vi "Test Harness.vi"() -> ()   [LabVIEW 2017, in "Command Handler.lvlib"]
uses:
  Command Handler.lvlib
  Command Handler/Command Handler.lvclass
  C:/Program Files (x86)/National Instruments/LabVIEW 2017/vi.lib/ActorFramework/Actor/Actor.lvclass
  <vilib>/ActorFramework/Message Enqueuer/Message Enqueuer.lvclass/Message Enqueuer.ctl
  Command Parents/Command.lvclass
  Command Handler Messages/Load Command Msg/Load Command Msg.lvclass/Load Command Msg.ctl
  Command Handler Messages/Execute Command Msg/Execute Command Msg.lvclass/Execute Command Msg.ctl
  Command Handler Messages/Execute Loaded Commands Msg/Execute Loaded Commands Msg.lvclass/Execute Loaded Commands Msg.ctl
  <vilib>/ActorFramework/Message Enqueuer/Enqueue.vi
  <vilib>/ActorFramework/Stop Msg/Stop Msg.lvclass
  C:/Program Files (x86)/National Instruments/LabVIEW 2017/vi.lib/ActorFramework/Message/Message.lvclass
  Command Handler Messages/Load Command Msg/Load Command Msg.lvclass
  Command Handler Messages/Execute Command Msg/Execute Command Msg.lvclass
  Command Handler Messages/Execute Loaded Command Msg/Execute Loaded Command Msg.lvclass
  Command Handler Messages/Execute Loaded Commands Msg/Execute Loaded Commands Msg.lvclass
  <vilib>/ActorFramework/Message Priority Queue/Priority Enqueue.vi
  <vilib>/ActorFramework/Actor/Actor.lvclass
  Command Handler Messages/Return Events Msg/Return Events Msg.lvclass
panel:
  in  "Commands Folder":path
  out "Last Error Time":timestamp
  in  "Enable Command Handling":bool
  in  "Disable Command Handling":bool
  in  "Reload":bool
  out "Last Handler Error":errorcluster
  in  "Commands":string(combo)
  in  "Run Loaded Commands":bool
  in  "Front (T) Back (F)":bool
  in  "Run Next Loaded Command":bool
  in  "Execute Command":bool
  in  "Add Command":bool
  out "Completed Commands":string[](array[string])
  out "Commands Completed":i32
  out "Loaded Commands":string[](array[string])
  out "Commands Loaded":i32
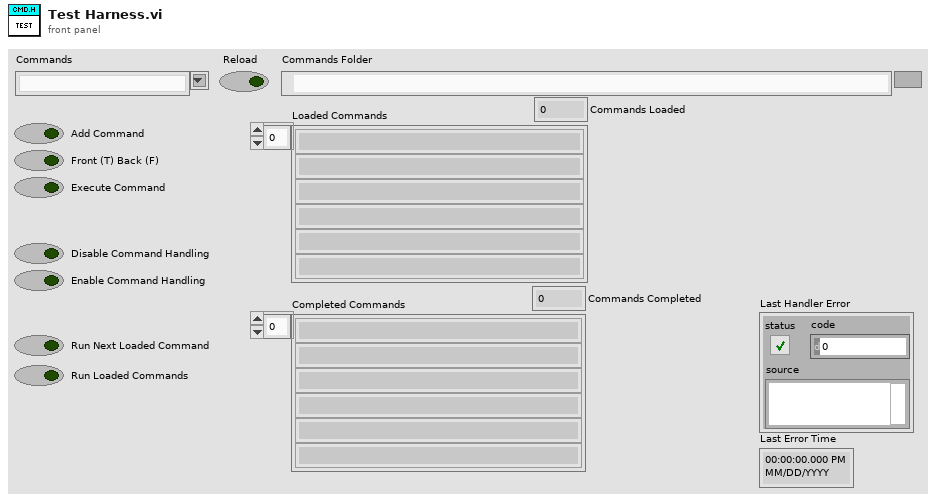
[diagram p1: front panel]
types:
  T1 = typedef "Command Handler.lvlib/Command Handler.lvclass/Event Cluster.ctl" = cluster{"Error Event":refnum<user-event>, "Command Done Event":refnum<user-event>, "Stopping Event":refnum<user-event>, "Data Update Event":refnum<user-event>}
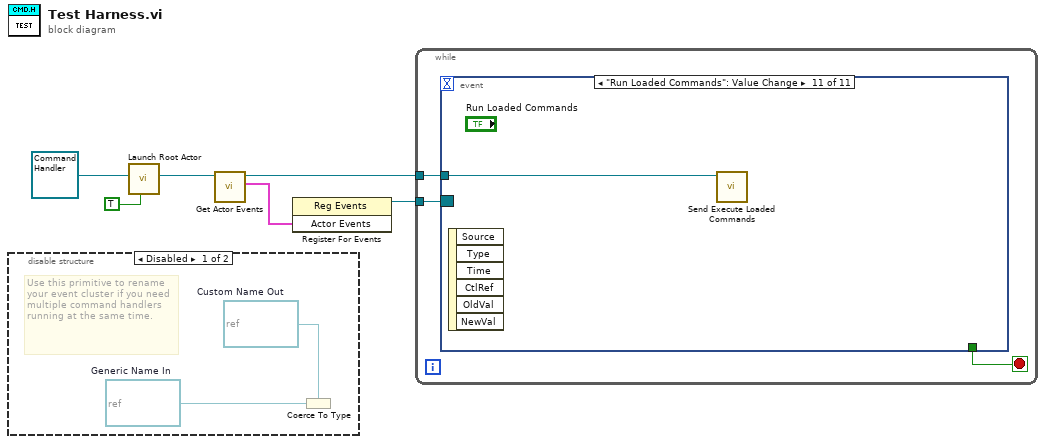
[diagram p0: block diagram]
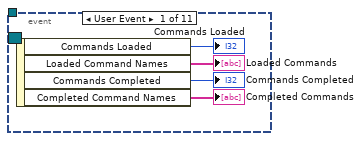
[diagram p3: hidden frame]
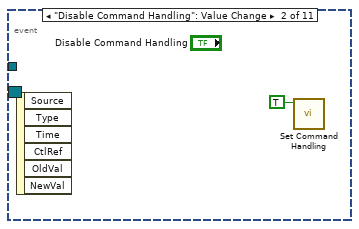
[diagram p4: hidden frame]
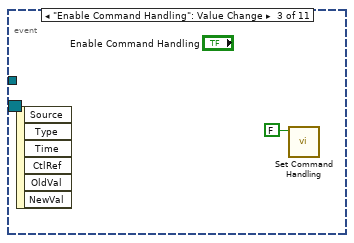
[diagram p5: hidden frame]
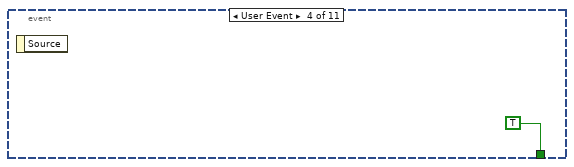
[diagram p6: hidden frame]
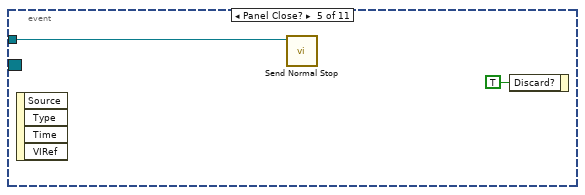
[diagram p7: hidden frame]
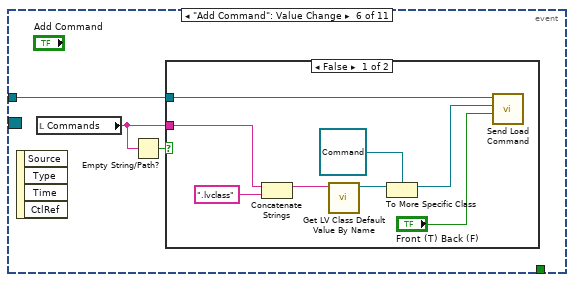
[diagram p8: hidden frame]
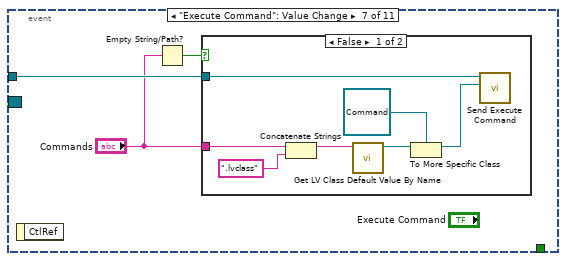
[diagram p10: hidden frame]
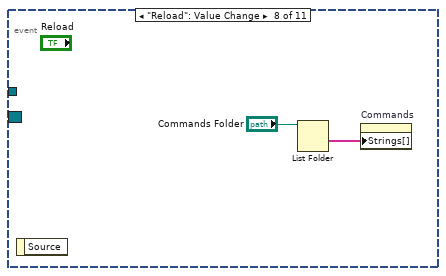
[diagram p12: hidden frame]
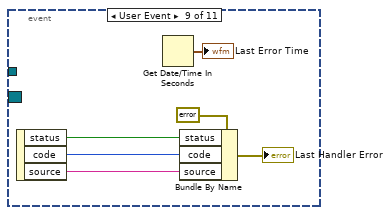
[diagram p13: hidden frame]
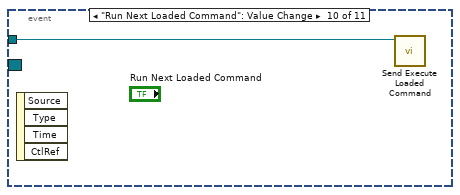
[diagram p14: hidden frame]
diagram:
  n1 = disable-structure shown="Disabled" {
    frame Disabled {
      w7 = refnum<user-event> refnum  # Custom Name Out
      w8 = refnum<user-event> refnum  # Generic Name In
      # "Use this primitive to rename your event cluster if you need multiple command handlers running at the same time."
      n2 = Coerce To Type(0:w8, 1:w7) -> ()  [unwired: 1 out]
    }
    frame Enabled {
    }
  }
  n3 = call <vilib>:"Launch Root Actor.vi"("Open Actor Core front panel? (F)"=TRUE, "Actor"=refnum<class "Command Handler.lvclass"> refnum ("Command Handler.lvlib:Command Handler.lvclass")) -> ("Actor's Enqueuer"=w1:refnum<class "Message Enqueuer.lvclass">)  [unwired: 8 in, 1 out]
  n4 = call "Get Actor Events.vi"("Message Enqueuer in"=w1) -> ("Actor Events"=w2:T1, "Message Enqueuer out"=w5:refnum<class "Message Enqueuer.lvclass">)  [unwired: 7 in, 2 out]
  n5 = register-events(w2) -> (reference out=w6:refnum<event-registration>)  [unwired: 2 in, 1 out]
  n6 = while {
    tunnel: w6 -> [w11]
    tunnel: w5 -> [w9]
    stop <- w10 stop-if-true
    n7 = event shown="[10] \"Run Loaded Commands\": Value Change" {
      selector: w11 -> [_ _ _ _ _ _ _ _ _ _ _]
      dyn-events: _ -> [_ _ _ _ _ _ _ _ _ _ _]
      timeout: _ -> [_ _ _ _ _ _ _ _ _ _ _]
      tunnel: [_ _ _ TRUE _ _ _ _ _ _ _] -> w10
      tunnel: w9 -> [_ _ _ _ w20 w23 w34 _ _ w50 w51]
      event User Event {
        n8 = event-data() -> ("Commands Loaded"=→"Commands Loaded":i32, "Loaded Command Names"=→"Loaded Commands":string[], "Commands Completed"=→"Commands Completed":i32, "Completed Command Names"=→"Completed Commands":string[])  [unwired: 1 in]
      }
      event "Disable Command Handling": Value Change {
        n9 = event-data() -> ()  [unwired: 1 in, 6 out]
        n10 = call "Set Command Handling.vi"("Disable Command Handling"=TRUE ("Command Handling Stopped")) -> ()  [unwired: 10 in, 1 out]
      }
      event "Enable Command Handling": Value Change {
        n11 = event-data() -> ()  [unwired: 1 in, 6 out]
        n12 = call "Set Command Handling.vi"("Disable Command Handling"=FALSE ("Command Handling Stopped")) -> ()  [unwired: 10 in, 1 out]
      }
      event User Event {
        n13 = event-data() -> ()  [unwired: 1 in, 1 out]
      }
      event Panel Close? {
        n14 = event-data() -> ()  [unwired: 1 in, 4 out]
        n15 = call <vilib>:"Send Normal Stop.vi"("Message Enqueuer"=w20) -> ()  [unwired: 10 in, 1 out]
        n16 = event-data("Discard?"=TRUE) -> ()  [unwired: 1 in, 1 out]
      }
      event "Add Command": Value Change {
        n17 = event-data() -> ()  [unwired: 1 in, 4 out]
        n18 = local read "Commands"() -> (w22:string)
        n19 = Empty String/Path?(string/path=w22) -> (empty?=w21:bool)
        n20 = case shown="False" w21 {
          tunnel: w23 -> [w31 _]
          tunnel: w22 -> [w24 _]
          frame False {
            n21 = Concatenate Strings(w24, ".lvclass" ("string")) -> (w26:string)
            n22 = call <vilib>:"Get LV Class Default Value By Name.vi"("class name"=w26) -> ("object"=w29:refnum<class>)  [unwired: 9 in, 1 out]
            n23 = To More Specific Class(target class=refnum<class "Command.lvclass"> refnum ("Command.lvclass"), reference=w29) -> (specific class reference=w28:refnum<class "Command.lvclass">)  [unwired: 1 in, 1 out]
            n24 = call "Send Load Command.vi"("Front (T) Back (F)"="Front (T) Back (F)", "Command In"=w28, "Message Enqueuer"=w31) -> ()  [unwired: 7 in, 2 out]
          }
          frame True {
          }
        }
      }
      event "Execute Command": Value Change {
        n25 = event-data() -> ()  [unwired: 1 in, 1 out]
        n26 = Empty String/Path?(string/path="Commands") -> (empty?=w33:bool)
        n27 = case shown="False" w33 {
          tunnel: w34 -> [w41 _]
          tunnel: "Commands" -> [w35 _]
          frame False {
            n28 = Concatenate Strings(w35, ".lvclass" ("string")) -> (w38:string)
            n29 = call <vilib>:"Get LV Class Default Value By Name.vi"("class name"=w38) -> ("object"=w40:refnum<class>)  [unwired: 9 in, 1 out]
            n30 = To More Specific Class(target class=refnum<class "Command.lvclass"> refnum ("Command.lvclass"), reference=w40) -> (specific class reference=w37:refnum<class "Command.lvclass">)  [unwired: 1 in, 1 out]
            n31 = call "Send Execute Command.vi"("Command"=w37, "Message Enqueuer"=w41) -> ()  [unwired: 8 in, 2 out]
          }
          frame True {
          }
        }
      }
      event "Reload": Value Change {
        n32 = event-data() -> ()  [unwired: 1 in, 1 out]
        n33 = List Folder(path="Commands Folder") -> (folder names=w43:string[])  [unwired: 3 in, 3 out]
        n34 = property on="Commands" class="CmbBox"("Strings[]"=w43) -> ()  [unwired: 2 in, 2 out]
      }
      event User Event {
        n35 = event-data() -> ("status"=w48:bool, "code"=w47:i32, "source"=w46:string)  [unwired: 1 in]
        n36 = Get Date/Time In Seconds() -> (seconds since 1Jan1904=→"Last Error Time":timestamp)
        n37 = Bundle By Name(cluster=errorcluster {"status"=FALSE, "code"=0, "source"=""} ("error constant"), "status"=w48, "code"=w47, "source"=w46) -> (→"Last Handler Error":errorcluster)
      }
      event "Run Next Loaded Command": Value Change {
        n38 = event-data() -> ()  [unwired: 1 in, 4 out]
        n39 = call "Send Execute Loaded Command.vi"("Message Enqueuer"=w50) -> ()  [unwired: 9 in, 2 out]
      }
      event "Run Loaded Commands": Value Change {
        n40 = event-data() -> ()  [unwired: 1 in, 6 out]
        n41 = call "Send Execute Loaded Commands.vi"("Message Enqueuer"=w51) -> ()  [unwired: 9 in, 2 out]
      }
    }
  }
